vi "auto_puke.vi"() -> ()   [LabVIEW 2012, in "Mecanum Drive.lvrbt"]
uses:
  Mecanum Drive.lvrbt
  <vilib>/NXT/Hardware/Plugins/Tetrix DC Motor/TetrixDCMotorAddress.ctl
  SubVIs/auto_drive_TYP.ctl
  <vilib>/FTC/FTC ControllerState.ctl
  <vilib>/FTC/FTC POVState.ctl
  <vilib>/NXT/Dual Mode Library/Waits/Wait_Num(msec).vi
  <vilib>/NXT/NXTIO Xnodes/NXTIONodeSubVIs/TETRIX IO Check Battery.vi
  <vilib>/NXT/NXTIO Xnodes/NXTIONodeSubVIs/TETRIX IO Move DC Motors.vi
  <vilib>/NXT/Dual Mode Library/Display/drawText.vi
  <vilib>/NXT/Subs/LVHSConnector.ctl
  <vilib>/NXT/NXTIO Xnodes/AddressXNode/NXTIOAddress.xnode
  <vilib>/NXT/NXTIO Xnodes/NXTIOXNode/NXTIO.xnode
  <vilib>/NXT/LegoClasses/BrickReference/BrickReference.lvclass
panel:
  out "Enabled":bool
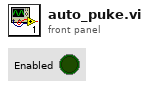
[diagram p1: front panel]
types:
  T1 = typedef "TetrixDCMotorAddress.ctl" = i32
  T2 = typedef "LVHSConnector.ctl" = refnum<class "BrickReference.lvclass">
  T3 = typedef "FTC ControllerState.ctl" = cluster{"Left X":i8, "Left Y":i8, "Right X":i8, "Right Y":i8, "Button Encoding 9-12":u8, "Button Encoding 1-8":u8, "POV":T4}
  T4 = typedef "FTC POVState.ctl" = i8
  T5 = cluster{"TetrixDCMotor":T1, "TetrixDCMotor 2":T1}
  T6 = typedef "auto_drive_TYP.ctl" = cluster{"Left X":i8, "Left Y":i8, "Right X":i8, "Power (100)":i8, "Wait (ms)":u32}
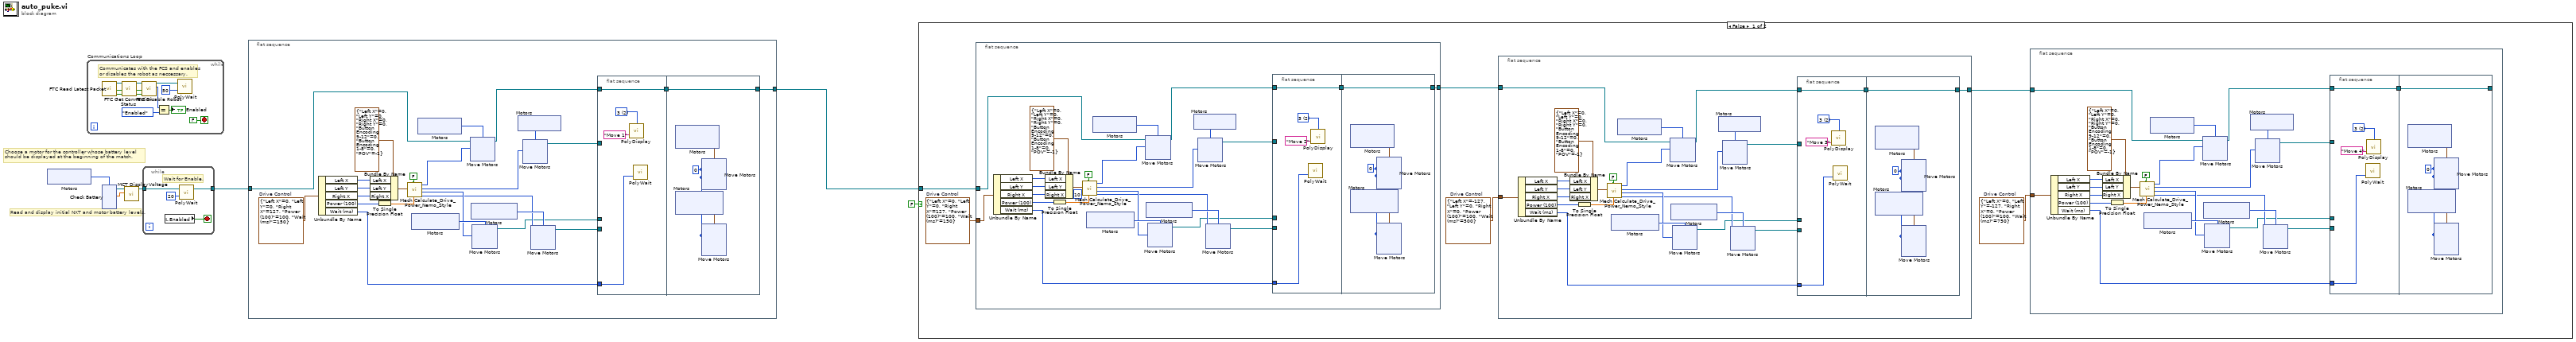
[diagram p0: block diagram]
diagram:
  # "Read and display initial NXT and motor battery levels."
  # "Choose a motor for the controller whose battery level \nshould be displayed at the beginning of the match."
  n1 = xnode "Motors"() -> ("Motor"=w4:T1)
  n2 = while "Communications Loop" {
    stop <- FALSE stop-if-true
    # "Communicates with the FCS and enables \nor disables the robot as neccessary."
    n3 = call <vilib>:"FTC Read Latest Packet.vi"() -> ("Packet Received?"=w17:bool, "Stopped?"=w16:bool, "NXT"=w19:T2)  [unwired: 6 in, 3 out]
    n4 = call <vilib>:"FTC Get Connection Status.vi"("Packet Received?"=w17, "Stopped?"=w16, "NXT"=w19) -> ("Online?"=w8:bool, "Stopped?"=w9:bool, "NXT"=w18:T2)  [unwired: 5 in]
    n5 = call <vilib>:"FTC Disable Robot.vi"("Online?"=w8, "Stopped?"=w9, "NXT"=w18) -> ("Enabled?"=w12:enum16{"Disabled", "Enabled"}, "NXT"=w14:T2)  [unwired: 3 in]
    n6 = Equal?(x=w12, y=enum16{"Disabled", "Enabled"}."Enabled") -> (x = y?=→"Enabled":bool)
    n7 = call-poly <vilib>:"PolyWait.vi"("Time (100 msec)"=u32 50 ("Time (msec)"), "NXT/EV3"=w14) -> ()  [unwired: 2 in, 1 out]
  }
  n8 = xnode "Check Battery"("Motors"=w4) -> ("Voltage 1"=w5:sgl, "NXT/EV3"=w7:T2)  [unwired: 1 in]
  n9 = call <vilib>:"MCT DisplayVoltage.vi"("Motor Voltage"=w5, "NXT"=w7) -> ("NXT"=w6:T2)  [unwired: 9 in]
  n10 = while {
    tunnel: [w21] -> w3
    tunnel: w6 -> [w20]
    stop <- w22 stop-if-true
    # "Wait for Enable."
    n11 = local read "Enabled"() -> (w22:bool)
    n12 = call-poly <vilib>:"PolyWait.vi"("Time (100 msec)"=u32 20 ("Time (msec)"), "NXT/EV3"=w20) -> ("NXT/EV3"=w21:T2)  [unwired: 2 in]
  }
  n13 = flat-sequence {
    tunnel: w3 -> [w25]
    tunnel: [w24] -> w2
    frame #0 {
      w26 = T6 {"Left X"=0, "Left Y"=0, "Right X"=127, "Power (100)"=100, "Wait (ms)"=150}  # Drive Control
      n14 = Unbundle By Name(w26) -> ("Left X"=w36:i8, "Left Y"=w35:i8, "Right X"=w34:i8, "Power (100)"=w28:i8, "Wait (ms)"=w29:u32)
      n15 = Bundle By Name(cluster=T3 {"Left X"=0, "Left Y"=0, "Right X"=0, "Right Y"=0, "Button Encoding 9-12"=0, "Button Encoding 1-8"=0, "POV"=-1} ("Controller State"), "Left X"=w36, "Left Y"=w35, "Right X"=w34) -> (w38:T3)
      n16 = To Single Precision Float(number=w28) -> (single precision float=w27:sgl)
      n17 = call "Mech Calculate_Drive_Power_Nemo_Style.vi"("Power"=w27, "Reverse"=FALSE, "Controller State"=w38) -> ("Right Rear Power"=w40:i8, "Right Front Power"=w41:i8, "Left Rear Power"=w42:i8, "Left Front Power"=w39:i8)  [unwired: 5 in]
      n18 = xnode ("Motors")() -> ("Motor"=w47:T1)
      n19 = xnode ("Motors")() -> ("Motor"=w44:T1)
      n20 = xnode ("Move Motors")("Power/Speed 1"=w39, "Motors"=w44, "NXT/EV3"=w25) -> ("NXT/EV3"=w33:T2)
      n21 = xnode ("Motors")() -> ("Motor"=w46:T1)
      n22 = xnode ("Move Motors")("Power/Speed 1"=w41, "Motors"=w47) -> ("NXT/EV3"=w30:T2)  [unwired: 1 in]
      n23 = xnode ("Motors")() -> ("Motor"=w45:T1)
      n24 = xnode ("Move Motors")("Power/Speed 1"=w42, "Motors"=w45) -> ("NXT/EV3"=w32:T2)  [unwired: 1 in]
      n25 = xnode ("Move Motors")("Power/Speed 1"=w40, "Motors"=w46) -> ("NXT/EV3"=w31:T2)  [unwired: 1 in]
      n26 = flat-sequence {
        tunnel: w33 -> [w52]
        tunnel: w32 -> [_]
        tunnel: w31 -> [_]
        tunnel: w30 -> [_]
        tunnel: w29 -> [w51]
        tunnel: [w52] -> w48
        tunnel: [w56] -> w24
        tunnel: w48 -> [w56]
        frame #0 {
          w49 = i16 2 items=["1", "2", "3", "4", "5", "6", "7", "8", "9", "10", "11", "12"] ("Line")
          n27 = call-poly <vilib>:"PolyDisplay.vi"("Text"="Move 1", "Line"=w49) -> ()  [unwired: 2 in, 1 out]
          n28 = call-poly <vilib>:"PolyWait.vi"("Time (100 msec)"=w51) -> ()  [unwired: 3 in, 1 out]
        }
        frame #1 {
          w53 = i8 0 ("Power/Speed 1")
          n29 = xnode "Motors"() -> ("Motor"=w55:cluster{"TetrixDCMotor":T1, "TetrixDCMotor":T1})
          n30 = xnode "Motors"() -> ("Motor"=w54:cluster{"TetrixDCMotor":T1, "TetrixDCMotor":T1})
          n31 = xnode "Move Motors"("Power/Speed 2"=w53, "Power/Speed 1"=w53, "Motors"=w55) -> ()  [unwired: 1 in, 1 out]
          n32 = xnode "Move Motors"("Power/Speed 2"=w53, "Power/Speed 1"=w53, "Motors"=w54) -> ()  [unwired: 1 in, 1 out]
        }
      }
    }
  }
  n33 = case shown="False" FALSE {
    tunnel: w2 -> [w111 _]
    frame False {
      w110 = T6 {"Left X"=-127, "Left Y"=0, "Right X"=0, "Power (100)"=100, "Wait (ms)"=500}  # Drive Control
      w108 = T6 {"Left X"=0, "Left Y"=-127, "Right X"=0, "Power (100)"=100, "Wait (ms)"=750}  # Drive Control
      w112 = T6 {"Left X"=0, "Left Y"=0, "Right X"=127, "Power (100)"=100, "Wait (ms)"=150}  # Drive Control
      n34 = flat-sequence {
        tunnel: w112 -> [w281]
        tunnel: w111 -> [w280]
        tunnel: [w279] -> w109
        frame #0 {
          n35 = Unbundle By Name(w281) -> ("Left X"=w291:i8, "Left Y"=w290:i8, "Right X"=w289:i8, "Power (100)"=w283:i8, "Wait (ms)"=w284:u32)
          n36 = Bundle By Name(cluster=T3 {"Left X"=0, "Left Y"=0, "Right X"=0, "Right Y"=0, "Button Encoding 9-12"=0, "Button Encoding 1-8"=0, "POV"=-1} ("Controller State"), "Left X"=w291, "Left Y"=w290, "Right X"=w289) -> (w293:T3)
          n37 = To Single Precision Float(number=w283) -> (single precision float=w282:sgl)
          n38 = call "Mech Calculate_Drive_Power_Nemo_Style.vi"("Power"=w282, "Reverse"=FALSE, "Deadband (10)"=i8 10, "Controller State"=w293) -> ("Right Rear Power"=w295:i8, "Right Front Power"=w296:i8, "Left Rear Power"=w297:i8, "Left Front Power"=w294:i8)  [unwired: 4 in]
          n39 = xnode ("Motors")() -> ("Motor"=w302:T1)
          n40 = xnode ("Motors")() -> ("Motor"=w299:T1)
          n41 = xnode ("Move Motors")("Power/Speed 1"=w294, "Motors"=w299, "NXT/EV3"=w280) -> ("NXT/EV3"=w288:T2)
          n42 = xnode ("Motors")() -> ("Motor"=w301:T1)
          n43 = xnode ("Move Motors")("Power/Speed 1"=w296, "Motors"=w302) -> ("NXT/EV3"=w285:T2)  [unwired: 1 in]
          n44 = xnode ("Motors")() -> ("Motor"=w300:T1)
          n45 = xnode ("Move Motors")("Power/Speed 1"=w297, "Motors"=w300) -> ("NXT/EV3"=w287:T2)  [unwired: 1 in]
          n46 = xnode ("Move Motors")("Power/Speed 1"=w295, "Motors"=w301) -> ("NXT/EV3"=w286:T2)  [unwired: 1 in]
          n47 = flat-sequence {
            tunnel: w288 -> [w307]
            tunnel: w287 -> [_]
            tunnel: w286 -> [_]
            tunnel: w285 -> [_]
            tunnel: w284 -> [w306]
            tunnel: [w307] -> w303
            tunnel: [w311] -> w279
            tunnel: w303 -> [w311]
            frame #0 {
              w305 = i16 2 items=["1", "2", "3", "4", "5", "6", "7", "8", "9", "10", "11", "12"] ("Line")
              n48 = call-poly <vilib>:"PolyWait.vi"("Time (100 msec)"=w306) -> ()  [unwired: 3 in, 1 out]
              n49 = call-poly <vilib>:"PolyDisplay.vi"("Text"="Move 2", "Line"=w305) -> ()  [unwired: 2 in, 1 out]
            }
            frame #1 {
              w308 = i8 0 ("Power/Speed 1")
              n50 = xnode "Motors"() -> ("Motor"=w310:cluster{"TetrixDCMotor":T1, "TetrixDCMotor":T1})
              n51 = xnode "Motors"() -> ("Motor"=w309:cluster{"TetrixDCMotor":T1, "TetrixDCMotor":T1})
              n52 = xnode "Move Motors"("Power/Speed 2"=w308, "Power/Speed 1"=w308, "Motors"=w310) -> ()  [unwired: 1 in, 1 out]
              n53 = xnode "Move Motors"("Power/Speed 2"=w308, "Power/Speed 1"=w308, "Motors"=w309) -> ()  [unwired: 1 in, 1 out]
            }
          }
        }
      }
      n54 = flat-sequence {
        tunnel: w110 -> [w197]
        tunnel: w109 -> [w196]
        tunnel: [w195] -> w107
        frame #0 {
          n55 = Unbundle By Name(w197) -> ("Left X"=w207:i8, "Left Y"=w206:i8, "Right X"=w205:i8, "Power (100)"=w199:i8, "Wait (ms)"=w200:u32)
          n56 = Bundle By Name(cluster=T3 {"Left X"=0, "Left Y"=0, "Right X"=0, "Right Y"=0, "Button Encoding 9-12"=0, "Button Encoding 1-8"=0, "POV"=-1} ("Controller State"), "Left X"=w207, "Left Y"=w206, "Right X"=w205) -> (w209:T3)
          n57 = To Single Precision Float(number=w199) -> (single precision float=w198:sgl)
          n58 = call "Mech Calculate_Drive_Power_Nemo_Style.vi"("Power"=w198, "Reverse"=FALSE, "Controller State"=w209) -> ("Right Rear Power"=w211:i8, "Right Front Power"=w212:i8, "Left Rear Power"=w213:i8, "Left Front Power"=w210:i8)  [unwired: 5 in]
          n59 = xnode ("Motors")() -> ("Motor"=w218:T1)
          n60 = xnode ("Motors")() -> ("Motor"=w215:T1)
          n61 = xnode ("Move Motors")("Power/Speed 1"=w210, "Motors"=w215, "NXT/EV3"=w196) -> ("NXT/EV3"=w204:T2)
          n62 = xnode ("Motors")() -> ("Motor"=w217:T1)
          n63 = xnode ("Move Motors")("Power/Speed 1"=w212, "Motors"=w218) -> ("NXT/EV3"=w201:T2)  [unwired: 1 in]
          n64 = xnode ("Motors")() -> ("Motor"=w216:T1)
          n65 = xnode ("Move Motors")("Power/Speed 1"=w213, "Motors"=w216) -> ("NXT/EV3"=w203:T2)  [unwired: 1 in]
          n66 = xnode ("Move Motors")("Power/Speed 1"=w211, "Motors"=w217) -> ("NXT/EV3"=w202:T2)  [unwired: 1 in]
          n67 = flat-sequence {
            tunnel: w204 -> [w223]
            tunnel: w203 -> [_]
            tunnel: w202 -> [_]
            tunnel: w201 -> [_]
            tunnel: w200 -> [w222]
            tunnel: [w223] -> w219
            tunnel: [w227] -> w195
            tunnel: w219 -> [w227]
            frame #0 {
              w220 = i16 2 items=["1", "2", "3", "4", "5", "6", "7", "8", "9", "10", "11", "12"] ("Line")
              n68 = call-poly <vilib>:"PolyDisplay.vi"("Text"="Move 3", "Line"=w220) -> ()  [unwired: 2 in, 1 out]
              n69 = call-poly <vilib>:"PolyWait.vi"("Time (100 msec)"=w222) -> ()  [unwired: 3 in, 1 out]
            }
            frame #1 {
              w224 = i8 0 ("Power/Speed 1")
              n70 = xnode "Motors"() -> ("Motor"=w226:cluster{"TetrixDCMotor":T1, "TetrixDCMotor":T1})
              n71 = xnode "Motors"() -> ("Motor"=w225:cluster{"TetrixDCMotor":T1, "TetrixDCMotor":T1})
              n72 = xnode "Move Motors"("Power/Speed 2"=w224, "Power/Speed 1"=w224, "Motors"=w226) -> ()  [unwired: 1 in, 1 out]
              n73 = xnode "Move Motors"("Power/Speed 2"=w224, "Power/Speed 1"=w224, "Motors"=w225) -> ()  [unwired: 1 in, 1 out]
            }
          }
        }
      }
      n74 = flat-sequence {
        tunnel: w108 -> [w114]
        tunnel: w107 -> [w113]
        frame #0 {
          n75 = Unbundle By Name(w114) -> ("Left X"=w124:i8, "Left Y"=w123:i8, "Right X"=w122:i8, "Power (100)"=w116:i8, "Wait (ms)"=w117:u32)
          n76 = Bundle By Name(cluster=T3 {"Left X"=0, "Left Y"=0, "Right X"=0, "Right Y"=0, "Button Encoding 9-12"=0, "Button Encoding 1-8"=0, "POV"=-1} ("Controller State"), "Left X"=w124, "Left Y"=w123, "Right X"=w122) -> (w126:T3)
          n77 = To Single Precision Float(number=w116) -> (single precision float=w115:sgl)
          n78 = call "Mech Calculate_Drive_Power_Nemo_Style.vi"("Power"=w115, "Reverse"=FALSE, "Controller State"=w126) -> ("Right Rear Power"=w128:i8, "Right Front Power"=w129:i8, "Left Rear Power"=w130:i8, "Left Front Power"=w127:i8)  [unwired: 5 in]
          n79 = xnode ("Motors")() -> ("Motor"=w135:T1)
          n80 = xnode ("Motors")() -> ("Motor"=w132:T1)
          n81 = xnode ("Move Motors")("Power/Speed 1"=w127, "Motors"=w132, "NXT/EV3"=w113) -> ("NXT/EV3"=w121:T2)
          n82 = xnode ("Motors")() -> ("Motor"=w134:T1)
          n83 = xnode ("Move Motors")("Power/Speed 1"=w129, "Motors"=w135) -> ("NXT/EV3"=w118:T2)  [unwired: 1 in]
          n84 = xnode ("Motors")() -> ("Motor"=w133:T1)
          n85 = xnode ("Move Motors")("Power/Speed 1"=w130, "Motors"=w133) -> ("NXT/EV3"=w120:T2)  [unwired: 1 in]
          n86 = xnode ("Move Motors")("Power/Speed 1"=w128, "Motors"=w134) -> ("NXT/EV3"=w119:T2)  [unwired: 1 in]
          n87 = flat-sequence {
            tunnel: w121 -> [w140]
            tunnel: w120 -> [_]
            tunnel: w119 -> [_]
            tunnel: w118 -> [_]
            tunnel: w117 -> [w139]
            tunnel: [w140] -> w136
            tunnel: [w144] -> _
            tunnel: w136 -> [w144]
            frame #0 {
              w138 = i16 2 items=["1", "2", "3", "4", "5", "6", "7", "8", "9", "10", "11", "12"] ("Line")
              n88 = call-poly <vilib>:"PolyWait.vi"("Time (100 msec)"=w139) -> ()  [unwired: 3 in, 1 out]
              n89 = call-poly <vilib>:"PolyDisplay.vi"("Text"="Move 4", "Line"=w138) -> ()  [unwired: 2 in, 1 out]
            }
            frame #1 {
              w141 = i8 0 ("Power/Speed 1")
              n90 = xnode "Motors"() -> ("Motor"=w143:cluster{"TetrixDCMotor":T1, "TetrixDCMotor":T1})
              n91 = xnode "Motors"() -> ("Motor"=w142:cluster{"TetrixDCMotor":T1, "TetrixDCMotor":T1})
              n92 = xnode "Move Motors"("Power/Speed 2"=w141, "Power/Speed 1"=w141, "Motors"=w143) -> ()  [unwired: 1 in, 1 out]
              n93 = xnode "Move Motors"("Power/Speed 2"=w141, "Power/Speed 1"=w141, "Motors"=w142) -> ()  [unwired: 1 in, 1 out]
            }
          }
        }
      }
    }
    frame True {
    }
  }
